vi "rpm_monitor.vi"() -> ()   [LabVIEW 2023]
uses:
  pico_scpi_labtool_labview_driver/scpi_driver/usbtmc_scpi_labtool.lvlib
panel:
  out "timestamp":dbl
  in  "On/Off Switch":bool
  in  "Digital Write Pin":u8 max=7 step=1
  out "rpm5":dbl
  out "rpm4":dbl
  out "rpm3":dbl
  out "rpm2":dbl
  out "rpm1":dbl
  out "rpm_new":dbl
  out "Meter":dbl(knob) scale=0.0..10000.0
  out "timer_diff (in ms)":dbl
  out "time_stamp":dbl
  out "count":dbl
  in  "stop":bool
  out "Waveform Chart":i32(graph)
  in  "Analog Read Pin":u8 max=7 step=1
  in  "VISA resource name in":refnum<visa-resource-name>="USB0::0xCAFE::0x4000::123456::INSTR"
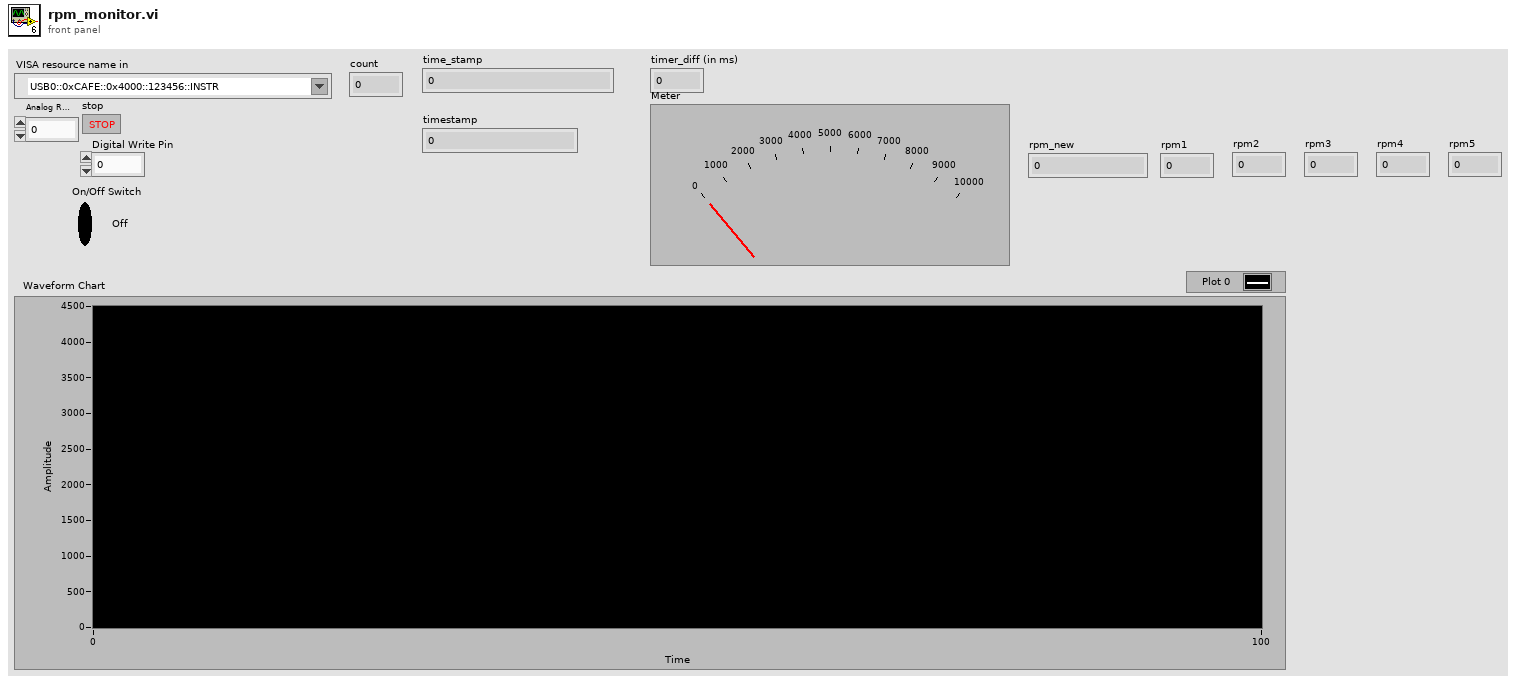
[diagram p1: front panel]
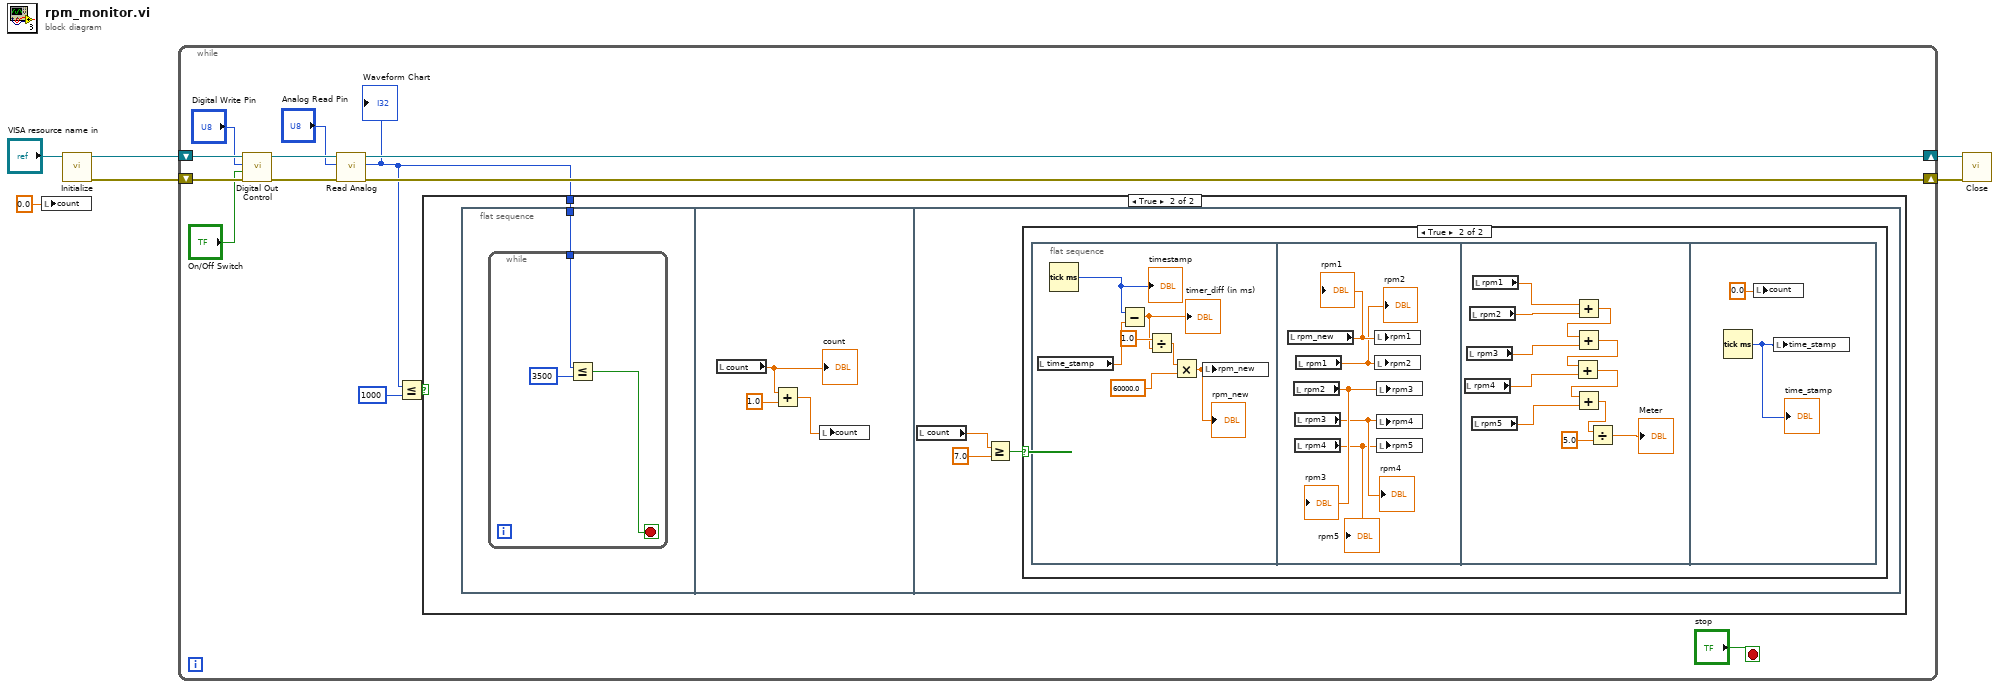
[diagram p0: block diagram]
diagram:
  n1 = local write "count"(0.0 ("count")) -> ()
  n2 = call "Initialize.vi"("VISA resource name in"="VISA resource name in") -> ("error out"=w4:errorcluster, "VISA resource name out"=w6:refnum<visa-resource-name>)  [unwired: 9 in]
  n3 = while {
    shift-right: [w19] -> w5
    shift-left: w6 -> [w16]
    shift-right: [w18] -> w3
    shift-left: w4 -> [w14]
    stop <- "stop" stop-if-true
    n4 = call "Digital Out Control.vi"("VISA resource name"=w16, "Pin"="Digital Write Pin", "Enable Pin (F: Off)"="On/Off Switch", "error in (no error)"=w14) -> ("VISA resource name out"=w15:refnum<visa-resource-name>, "error out"=w13:errorcluster)  [unwired: 5 in]
    n5 = call "Read Analog.vi"("error in (no error)"=w13, "Pin"="Analog Read Pin", "VISA resource name"=w15) -> ("error out"=w18:errorcluster, "analog out"=w7:i32, "VISA resource name out"=w19:refnum<visa-resource-name>)  [unwired: 6 in]
    "Waveform Chart" <- w7
    n6 = Less Or Equal?(x=w7, y=1000) -> (x <= y?=w8:bool)
    n7 = case shown="True" w8 {
      tunnel: w7 -> [_ w20]
      frame False {
      }
      frame True {
        n8 = flat-sequence {
          tunnel: w20 -> [w21]
          frame #0 {
            n9 = while {
              tunnel: w21 -> [w24]
              stop <- w22 stop-if-true
              n10 = Less Or Equal?(x=w24, y=3500) -> (x <= y?=w22:bool)
            }
          }
          frame #1 {
            n11 = local read "count"() -> (w27:dbl)
            "count" <- w27
            n12 = Add(x=w27, y=1.0) -> (x+y=w26:dbl)
            n13 = local write "count"(w26) -> ()
          }
          frame #2 {
            n14 = local read "count"() -> (w29:dbl)
            n15 = Greater Or Equal?(x=w29, y=7.0) -> (x >= y?=w30:bool)
            n16 = case shown="True" w30 {
              frame False {
              }
              frame True {
                n17 = flat-sequence {
                  frame #0 {
                    n18 = local read "time_stamp"() -> (w37:dbl)
                    n19 = Tick Count (ms)() -> (millisecond timer value=w34:u32)
                    "timestamp" <- w34
                    n20 = Subtract(x=w34, y=w37) -> (x-y=w32:dbl)
                    "timer_diff (in ms)" <- w32
                    n21 = Divide(x=1.0, y=w32) -> (x/y=w31:dbl)
                    n22 = Multiply(x=w31, y=60000.0) -> (x*y=w35:dbl)
                    "rpm_new" <- w35
                    n23 = local write "rpm_new"(w35) -> ()
                  }
                  frame #1 {
                    n24 = local read "rpm_new"() -> (w42:dbl)
                    "rpm1" <- w42
                    n25 = local read "rpm2"() -> (w40:dbl)
                    "rpm3" <- w40
                    n26 = local read "rpm3"() -> (w39:dbl)
                    "rpm4" <- w39
                    n27 = local read "rpm4"() -> (w38:dbl)
                    "rpm5" <- w38
                    n28 = local read "rpm1"() -> (w41:dbl)
                    "rpm2" <- w41
                    n29 = local write "rpm1"(w42) -> ()
                    n30 = local write "rpm2"(w41) -> ()
                    n31 = local write "rpm3"(w40) -> ()
                    n32 = local write "rpm4"(w39) -> ()
                    n33 = local write "rpm5"(w38) -> ()
                  }
                  frame #2 {
                    n34 = local read "rpm4"() -> (w48:dbl)
                    n35 = local read "rpm3"() -> (w50:dbl)
                    n36 = local read "rpm2"() -> (w52:dbl)
                    n37 = local read "rpm5"() -> (w46:dbl)
                    n38 = local read "rpm1"() -> (w53:dbl)
                    n39 = Add(x=w53, y=w52) -> (x+y=w51:dbl)
                    n40 = Add(x=w51, y=w50) -> (x+y=w49:dbl)
                    n41 = Add(x=w49, y=w48) -> (x+y=w47:dbl)
                    n42 = Add(x=w47, y=w46) -> (x+y=w45:dbl)
                    n43 = Divide(x=w45, y=5.0) -> (x/y=→"Meter":dbl)
                  }
                  frame #3 {
                    n44 = Tick Count (ms)() -> (millisecond timer value=w54:u32)
                    "time_stamp" <- w54
                    n45 = local write "count"(0.0 ("count")) -> ()
                    n46 = local write "time_stamp"(w54) -> ()
                  }
                }
              }
            }
          }
        }
      }
    }
  }
  n47 = call "Close.vi"("error in (no error)"=w3, "VISA resource name"=w5) -> ()  [unwired: 10 in]
